vi "Cycling_No_DAQ_Tasks_RT - cOver100.vi"() -> ()   [LabVIEW 2020]
uses:
  Device-Interface-Layer/stop button3.vi
  Device-Interface-Layer/stop button2.vi
  Device-Interface-Layer/stop button1.vi
panel:
  out "Battery 1 Temp":dbl(graph)
  out "Battery 1 Strain":dbl(graph)
  out "Battery 1 Voltage":dbl(graph)
  out "Battery 1 Current":dbl(graph)
  out "Battery 2 Temp":dbl(graph)
  out "Battery 2 Strain":dbl(graph)
  out "Battery 2 Voltage":dbl(graph)
  out "Battery 2 Current":dbl(graph)
  out "Battery 3 Current":dbl(graph)
  out "Battery 3 Voltage":dbl(graph)
  out "Battery 3 Strain":dbl(graph)
  out "Boolean":bool=TRUE
  out "Battery 3 Temp":dbl(graph)
  out "PS Visa Out 3":refnum<visa-resource-name>
  out "PS error out 3":errorcluster
  in  "PS error in 3":errorcluster caption="PS error in (no error)"
  out "PS Visa Out 2":refnum<visa-resource-name>
  out "PS error out 2":errorcluster
  in  "PS error in 2":errorcluster caption="PS error in (no error)"
  out "PS error out":errorcluster
  out "PS Visa Out":refnum<visa-resource-name>
  in  "PS error in":errorcluster caption="PS error in (no error)"
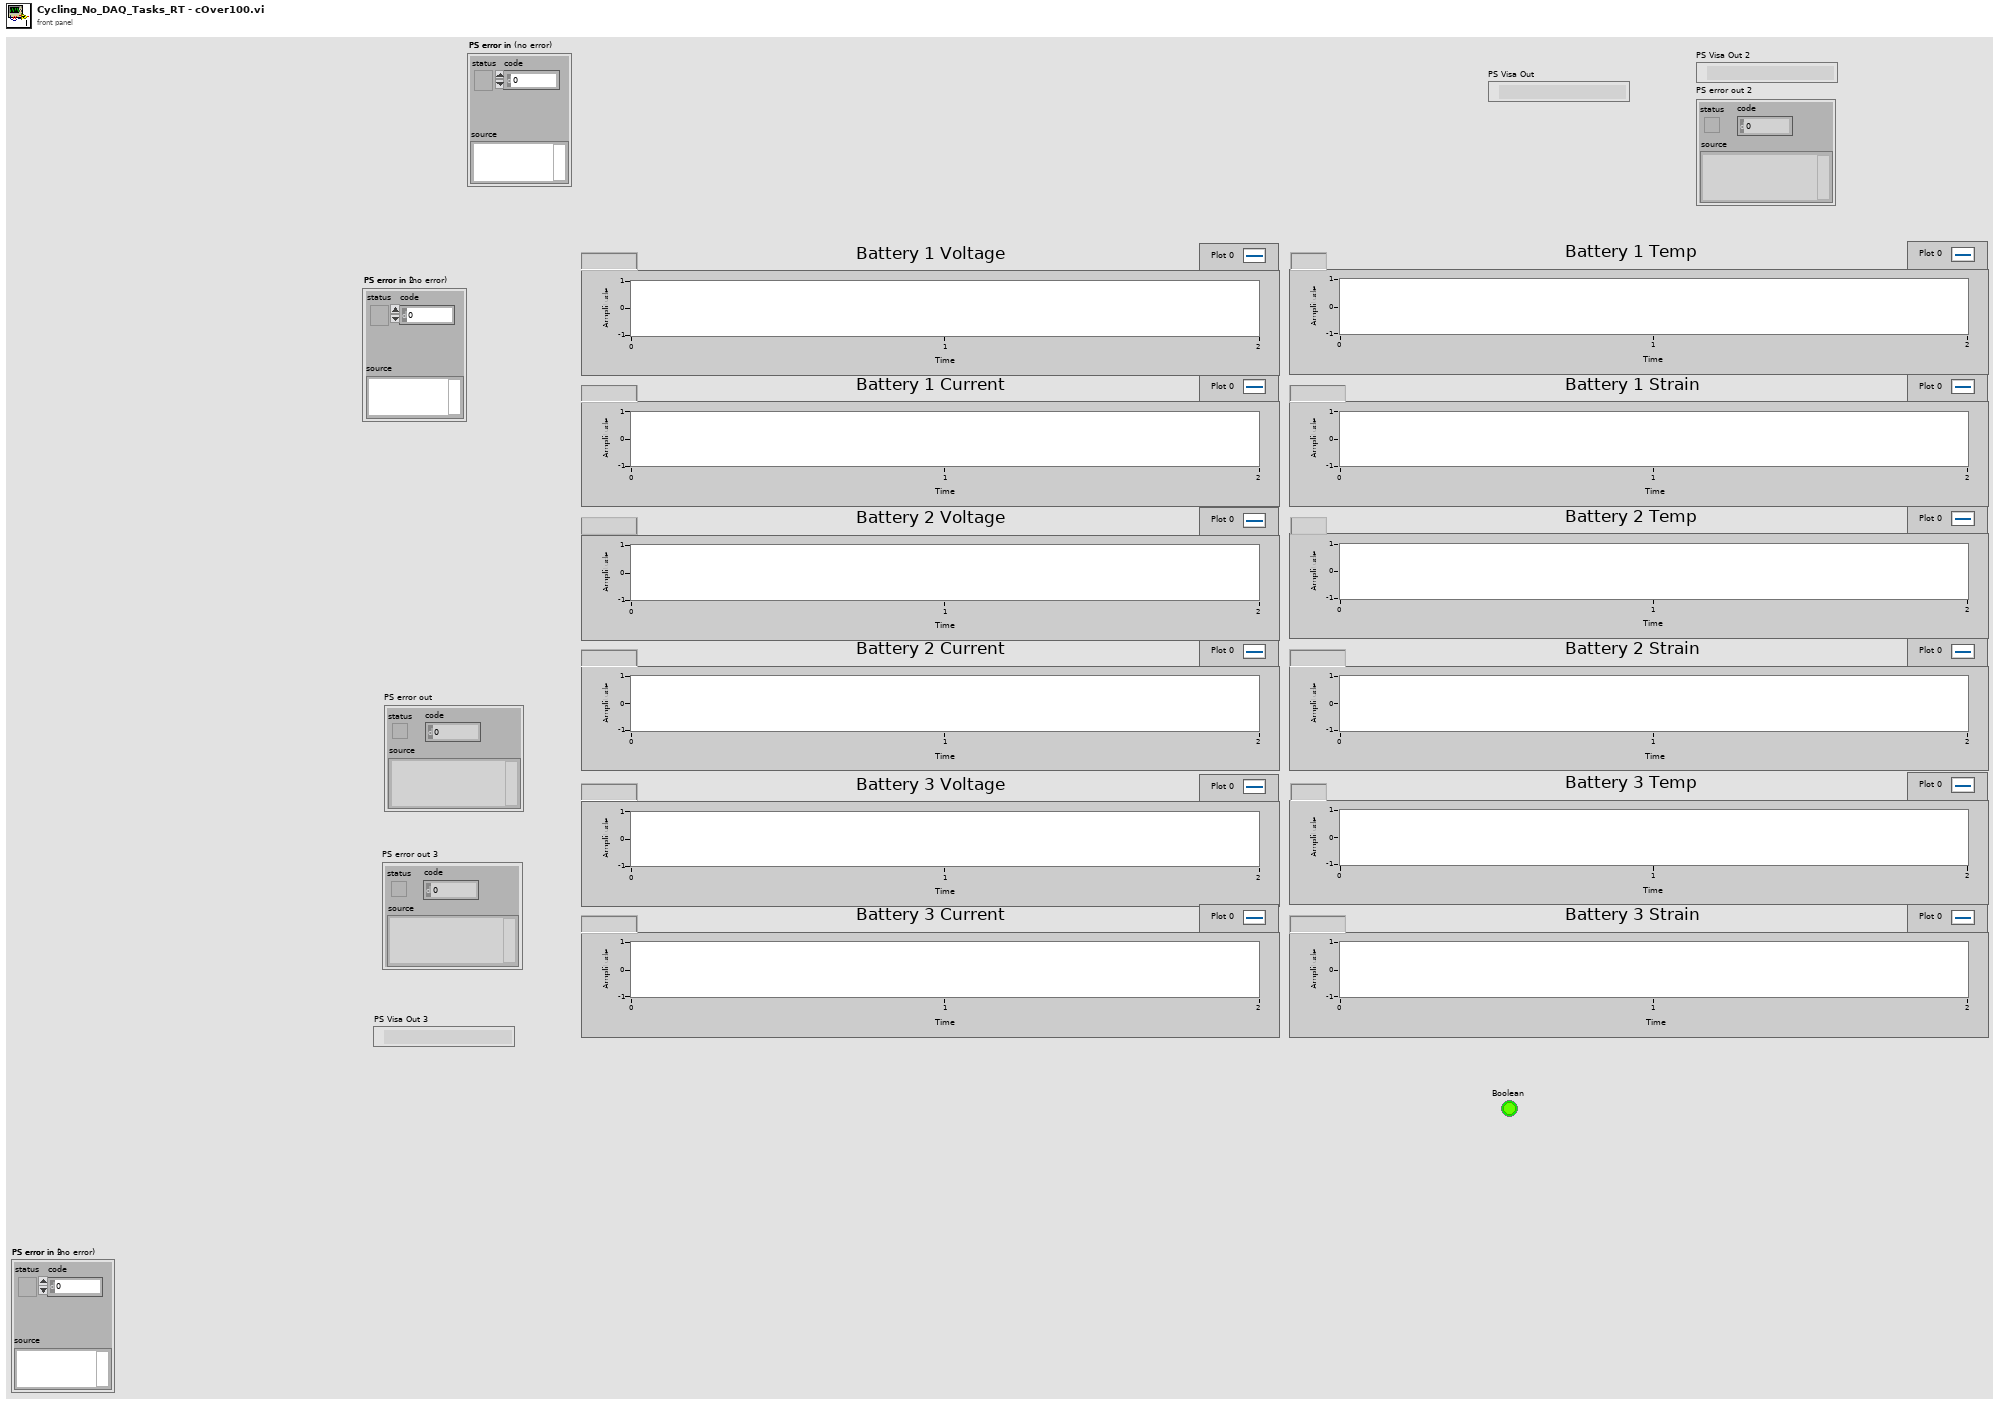
[diagram p1: front panel]
types:
  T1 = enum16{"\"30Q\"", "\"40T\"", "\"2P30Q\"", "\"3P30Q\"", "\"Nissan Leaf\""}
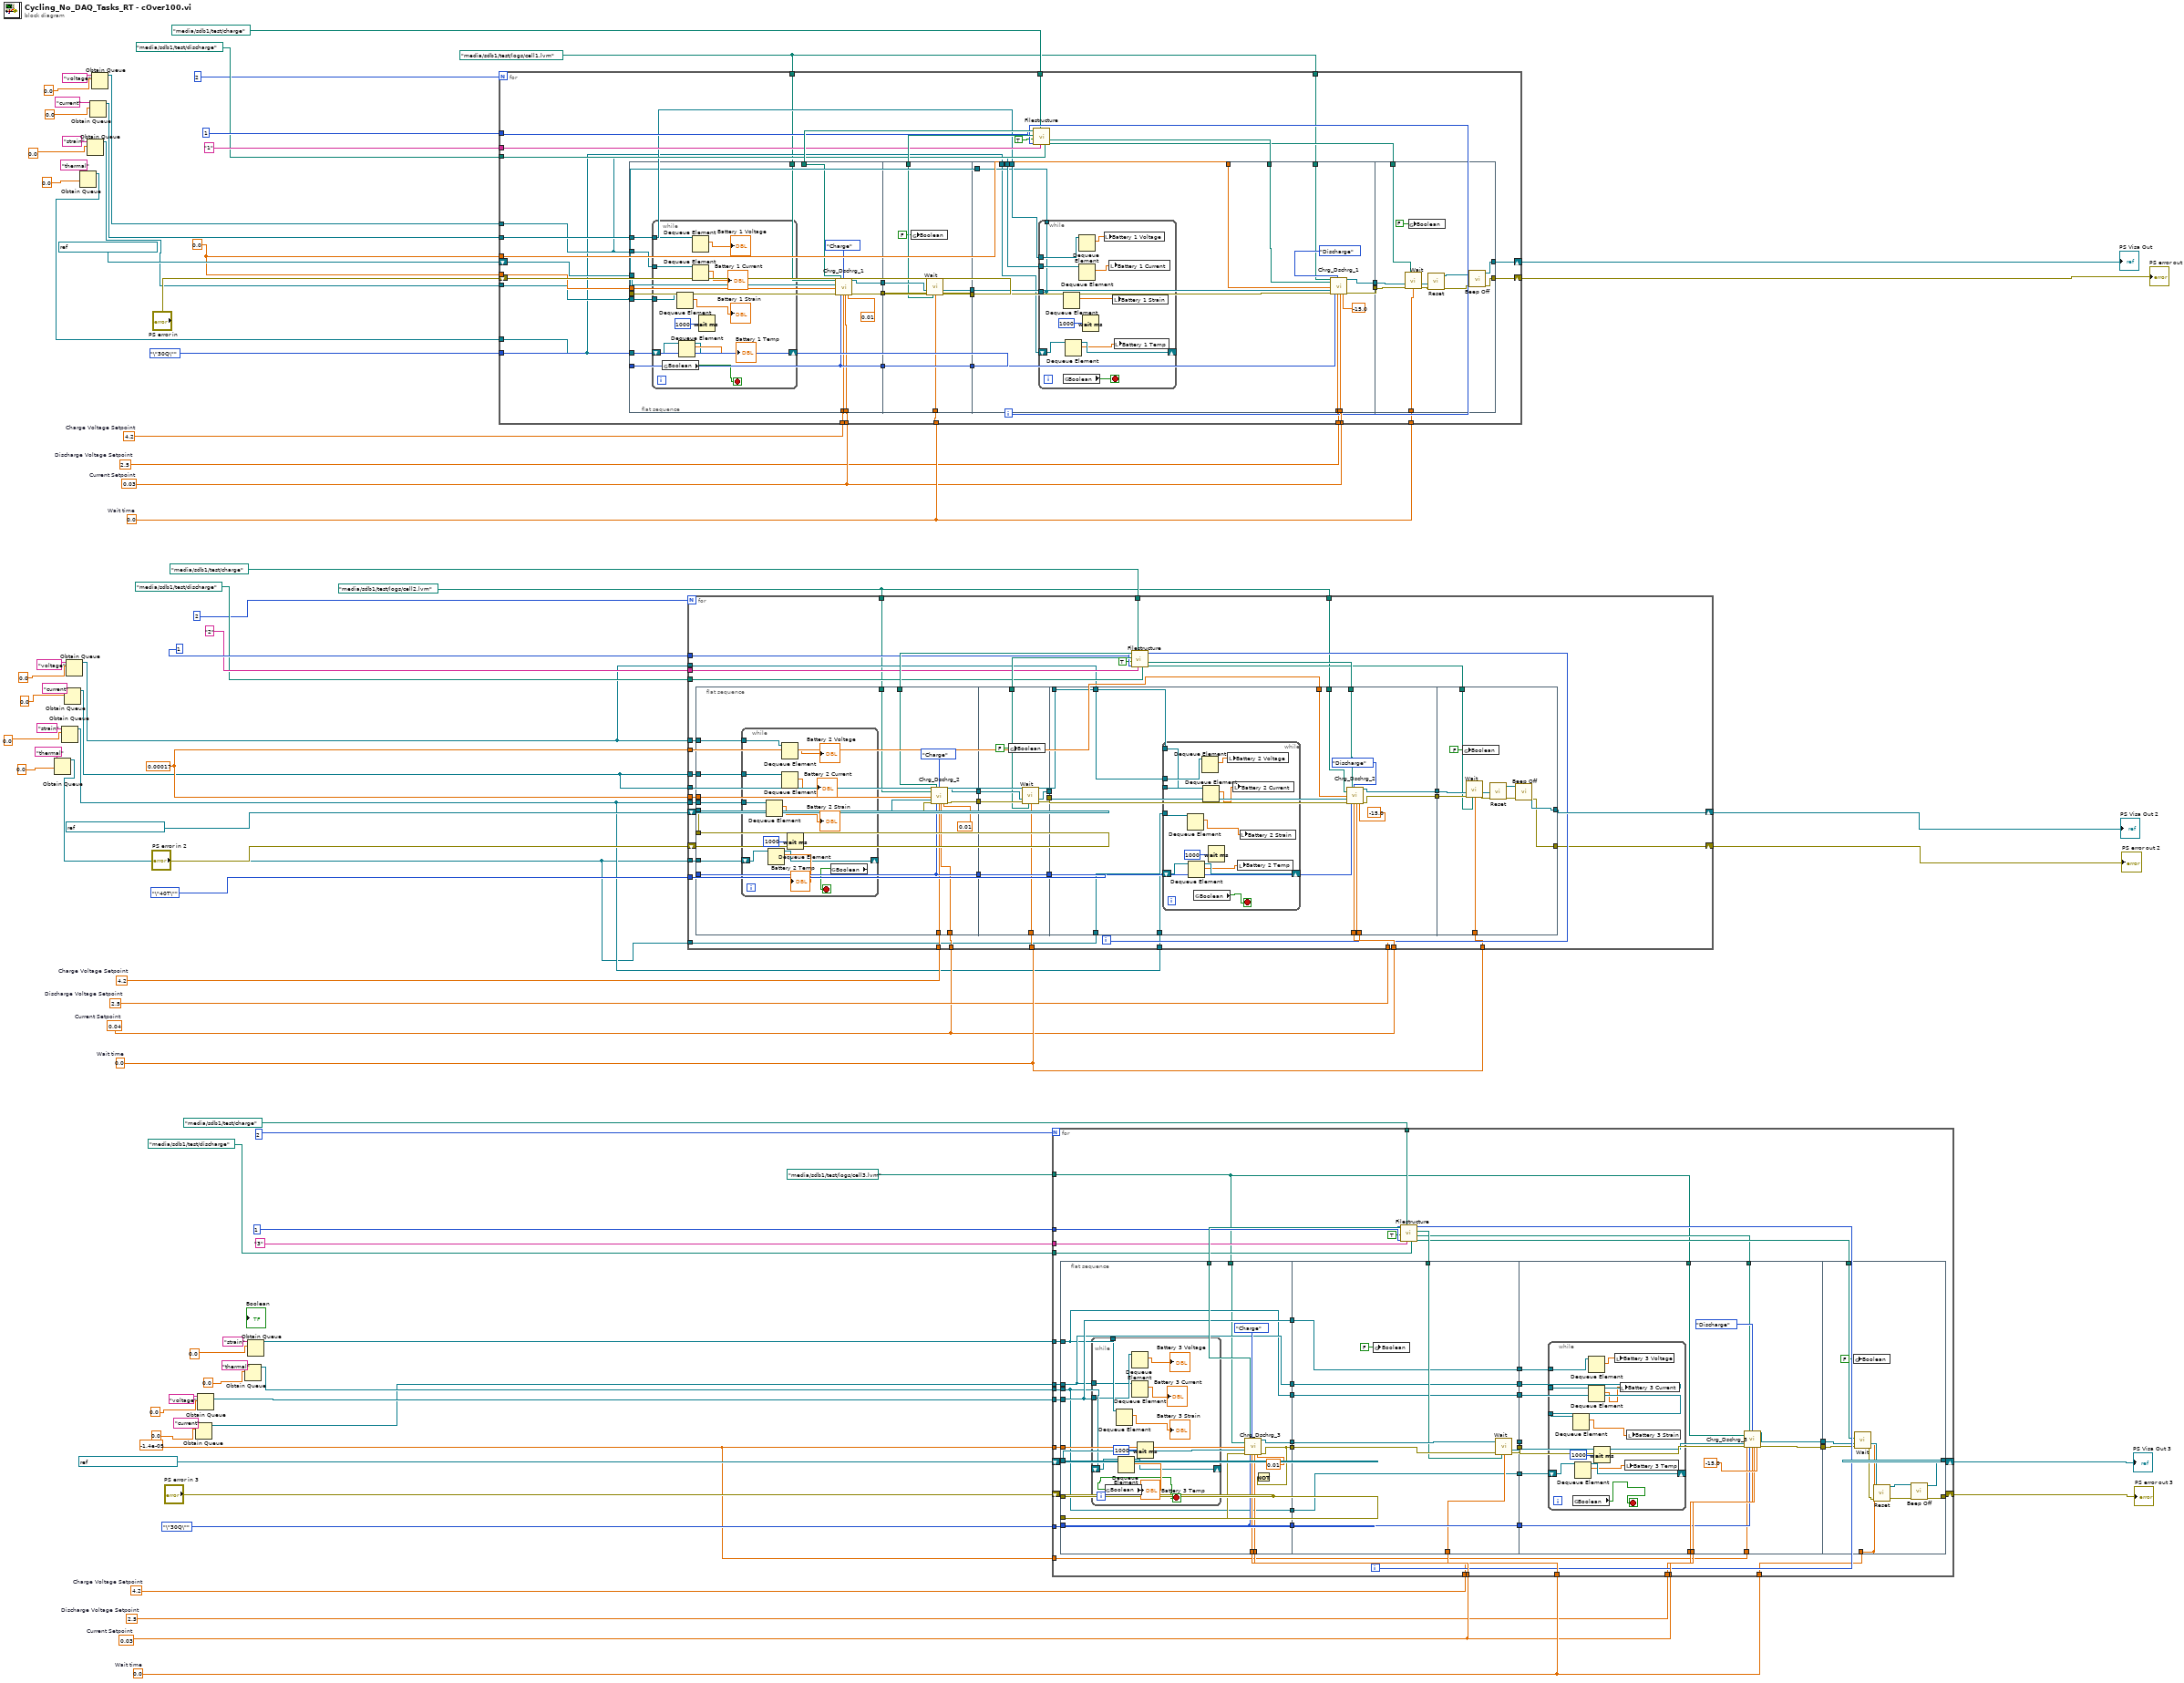
[diagram p0: block diagram]
diagram:
  w2 = path "/media/sdb1/test/logs/cell2.lvm" ("Error log filepath")
  w3 = path "/media/sdb1/test/logs/cell1.lvm" ("Error log filepath")
  w6 = -1.4e-05 ("Strain Offset")
  w41 = 0.00017 ("Strain Offset")
  w42 = 2.5  # Discharge Voltage Setpoint
  w45 = 0.0  # Wait time
  w43 = 0.03  # Current Setpoint
  w44 = 4.2  # Charge Voltage Setpoint
  w48 = 2.5  # Discharge Voltage Setpoint
  w49 = 0.0  # Wait time
  w47 = 0.04  # Current Setpoint
  w46 = 4.2  # Charge Voltage Setpoint
  w50 = 2.5  # Discharge Voltage Setpoint
  w53 = 0.0 ("Strain Offset")
  w54 = 0.0  # Wait time
  w52 = 0.03  # Current Setpoint
  w51 = 4.2  # Charge Voltage Setpoint
  n1 = Obtain Queue(name (unnamed)="thermal", element data type=0.0) -> (queue out=w7:refnum<queue>)  [unwired: 3 in, 2 out]
  n2 = Obtain Queue(name (unnamed)="strain", element data type=0.0) -> (queue out=w8:refnum<queue>)  [unwired: 3 in, 2 out]
  n3 = Obtain Queue(name (unnamed)="current", element data type=0.0) -> (queue out=w9:refnum<queue>)  [unwired: 3 in, 2 out]
  n4 = Obtain Queue(name (unnamed)="voltage", element data type=0.0) -> (queue out=w10:refnum<queue>)  [unwired: 3 in, 2 out]
  n5 = Obtain Queue(name (unnamed)="thermal", element data type=0.0) -> (queue out=w11:refnum<queue>)  [unwired: 3 in, 2 out]
  n6 = Obtain Queue(name (unnamed)="strain", element data type=0.0) -> (queue out=w12:refnum<queue>)  [unwired: 3 in, 2 out]
  n7 = Obtain Queue(name (unnamed)="current", element data type=0.0) -> (queue out=w13:refnum<queue>)  [unwired: 3 in, 2 out]
  n8 = Obtain Queue(name (unnamed)="voltage", element data type=0.0) -> (queue out=w14:refnum<queue>)  [unwired: 3 in, 2 out]
  n9 = Obtain Queue(name (unnamed)="current", element data type=0.0) -> (queue out=w33:refnum<queue>)  [unwired: 3 in, 2 out]
  n10 = Obtain Queue(name (unnamed)="voltage", element data type=0.0) -> (queue out=w34:refnum<queue>)  [unwired: 3 in, 2 out]
  n11 = Obtain Queue(name (unnamed)="thermal", element data type=0.0) -> (queue out=w39:refnum<queue>)  [unwired: 3 in, 2 out]
  n12 = Obtain Queue(name (unnamed)="strain", element data type=0.0) -> (queue out=w37:refnum<queue>)  [unwired: 3 in, 2 out]
  n13 = for {
    N: 2 ("Number of Cycles") -> [_]
    tunnel: T1."\"30Q\"" ("Battery Type") -> [w111]
    tunnel: w51 -> [w110]
    tunnel: w52 -> [w109]
    tunnel: w54 -> [w97]
    shift-right: [w88] -> w81
    shift-left: refnum<visa-resource-name> "TCPIP0::192.168.0.246::inst0::INSTR" ("PS VISA in") -> [w113]
    shift-right: [w87] -> w82
    shift-left: "PS error in" -> [w112]
    tunnel: 1 ("Starting Cycle") -> [w103]
    tunnel: "1" ("Batteryname") -> [w101]
    tunnel: path "/media/sdb1/test/discharge" ("Discharge filepath") -> [w100]
    tunnel: path "/media/sdb1/test/charge" ("Charge filepath") -> [w99]
    tunnel: w54 -> [w98]
    tunnel: w53 -> [w96]
    tunnel: w53 -> [w95]
    tunnel: w52 -> [w94]
    tunnel: w50 -> [w93]
    tunnel: w14 -> [w92]
    tunnel: w13 -> [w91]
    tunnel: w12 -> [w90]
    tunnel: w11 -> [w89]
    tunnel: w3 -> [w86]
    tunnel: w3 -> [w85]
    i -> [w104]
    n14 = flat-sequence {
      tunnel: w113 -> [w131]
      tunnel: w112 -> [w132]
      tunnel: w111 -> [w133]
      tunnel: w110 -> [w128]
      tunnel: [w135] -> w121
      tunnel: [w127] -> w120
      tunnel: [w133] -> w119
      tunnel: w108 -> [w136]
      tunnel: w96 -> [w130]
      tunnel: w94 -> [w129]
      tunnel: w92 -> [w126]
      tunnel: w91 -> [w125]
      tunnel: w90 -> [w124]
      tunnel: w89 -> [w123]
      tunnel: w86 -> [w122]
      tunnel: w121 -> [w155]
      tunnel: w120 -> [w154]
      tunnel: [w151] -> w118
      tunnel: [w152] -> w117
      tunnel: w119 -> [w156]
      tunnel: [w156] -> w116
      tunnel: w107 -> [w153]
      tunnel: w97 -> [w150]
      tunnel: w118 -> [w167]
      tunnel: w117 -> [w168]
      tunnel: w116 -> [w169]
      tunnel: w93 -> [w170]
      tunnel: w109 -> [w171]
      tunnel: w106 -> [w166]
      tunnel: [w164] -> w115
      tunnel: [w163] -> w114
      tunnel: w95 -> [w162]
      tunnel: w92 -> [w161]
      tunnel: w91 -> [w160]
      tunnel: w90 -> [w159]
      tunnel: w89 -> [w158]
      tunnel: w85 -> [w157]
      tunnel: w105 -> [w189]
      tunnel: w115 -> [w194]
      tunnel: w114 -> [w193]
      tunnel: w98 -> [w190]
      tunnel: [w185] -> w88
      tunnel: [w184] -> w87
      frame #0 {
        n15 = while {
          shift-right: [w146] -> _
          shift-left: w123 -> [w145]
          tunnel: w125 -> [w143]
          tunnel: w126 -> [w140]
          tunnel: w124 -> [w139]
          stop <- w138 stop-if-true
          n16 = global read "stop button1.vi" "Boolean"() -> (w138:bool)
          n17 = Dequeue Element(queue=w139) -> (element=→"Battery 1 Strain":dbl)  [unwired: 2 in, 3 out]
          n18 = Dequeue Element(queue=w145) -> (queue out=w146:refnum<queue>, element=→"Battery 1 Temp":dbl)  [unwired: 2 in, 2 out]
          n19 = Dequeue Element(queue=w140) -> (element=→"Battery 1 Voltage":dbl)  [unwired: 2 in, 3 out]
          n20 = Dequeue Element(queue=w143) -> (element=→"Battery 1 Current":dbl)  [unwired: 2 in, 3 out]
          n21 = Wait (ms)(milliseconds to wait=1000) -> ()  [unwired: 1 out]
        }
        n22 = call "Chrg_Dschrg_1.vi"("Error log filepath"=w122, "Strain Offset"=w130, "PS VISA in"=w131, "PS error in"=w132, "CyclePath"=w136, "Battery Type"=w133, "Charge/discharge"=enum8{"Charge", "Discharge"}."Charge", "Charge/Discharge Voltage Setpoint"=w128, "Current Setpoint"=w129, "Current Cutoff"=0.01) -> ("PS VISA out"=w135:refnum<visa-resource-name>, "PS error out"=w127:errorcluster)  [unwired: 8 in]
      }
      frame #1 {
        n23 = global write "stop button1.vi" "Boolean"(FALSE ("Boolean")) -> ()
        n24 = call "Wait.vi"("PS VISA in"=w155, "PS error in"=w154, "Wait Filepath"=w153, "Wait time"=w150) -> ("PS Visa Out"=w151:refnum<visa-resource-name>, "PS error out"=w152:errorcluster)  [unwired: 10 in]
      }
      frame #2 {
        n25 = while {
          shift-right: [w182] -> _
          shift-left: w158 -> [w181]
          tunnel: [w174] -> _
          tunnel: w160 -> [w180]
          tunnel: w161 -> [w175]
          tunnel: w159 -> [w174]
          stop <- w173 stop-if-true
          n26 = Dequeue Element(queue=w174) -> (element=w177:dbl)  [unwired: 2 in, 3 out]
          n27 = global read "stop button1.vi" "Boolean"() -> (w173:bool)
          n28 = Dequeue Element(queue=w181) -> (queue out=w182:refnum<queue>, element=w176:dbl)  [unwired: 2 in, 2 out]
          n29 = Dequeue Element(queue=w175) -> (element=w179:dbl)  [unwired: 2 in, 3 out]
          n30 = Dequeue Element(queue=w180) -> (element=w178:dbl)  [unwired: 2 in, 3 out]
          n31 = Wait (ms)(milliseconds to wait=1000) -> ()  [unwired: 1 out]
          n32 = local write "Battery 1 Voltage"(w179) -> ()
          n33 = local write "Battery 1 Current"(w178) -> ()
          n34 = local write "Battery 1 Strain"(w177) -> ()
          n35 = local write "Battery 1 Temp"(w176) -> ()
        }
        n36 = call "Chrg_Dschrg_1.vi"("Error log filepath"=w157, "Strain Offset"=w162, "PS VISA in"=w167, "PS error in"=w168, "CyclePath"=w166, "Battery Type"=w169, "Charge/discharge"=enum8{"Charge", "Discharge"}."Discharge", "Charge/Discharge Voltage Setpoint"=w170, "Current Setpoint"=w171, "Current Cutoff"=-15.0) -> ("PS VISA out"=w164:refnum<visa-resource-name>, "PS error out"=w163:errorcluster)  [unwired: 8 in]
      }
      frame #3 {
        n37 = call "Wait.vi"("PS VISA in"=w194, "PS error in"=w193, "Wait Filepath"=w189, "Wait time"=w190) -> ("PS Visa Out"=w192:refnum<visa-resource-name>, "PS error out"=w191:errorcluster)  [unwired: 10 in]
        n38 = global write "stop button1.vi" "Boolean"(FALSE ("Boolean")) -> ()
        n39 = call "Reset.vi"("error in"=w191, "VISA resource name"=w192) -> ("error out"=w186:errorcluster, "VISA resource name out"=w187:refnum<visa-resource-name>)  [unwired: 8 in]
        n40 = call "Beep Off.vi"("error in"=w186, "VISA resource name"=w187) -> ("error out"=w184:errorcluster, "VISA resource name out"=w185:refnum<visa-resource-name>)  [unwired: 8 in]
      }
    }
    n41 = call "Filestructure.vi"("Discharge filepath"=w100, "Batteryname"=w101, "Charge filepath"=w99, "For loop i"=w104, "In for loop"=TRUE, "Starting Cycle"=w103) -> ("DischargeWaitPath"=w105:path, "DischargeCyclePath"=w106:path, "ChargeWaitPath"=w107:path, "ChargeCyclePath"=w108:path)  [unwired: 1 in, 1 out]
  }
  "PS error out" <- w82
  "PS Visa Out" <- w81
  n42 = for {
    N: 2 ("Number of Cycles") -> [_]
    tunnel: T1."\"40T\"" ("Battery Type") -> [w225]
    tunnel: w47 -> [w224]
    tunnel: w47 -> [w223]
    shift-right: [w218] -> w71
    shift-left: refnum<visa-resource-name> "TCPIP0::192.168.0.247::inst0::INSTR" ("PS VISA in") -> [w227]
    shift-right: [w211] -> w72
    shift-left: "PS error in 2" -> [w226]
    tunnel: 1 ("Starting Cycle") -> [w216]
    tunnel: "2" ("Batteryname 2") -> [w214]
    tunnel: path "/media/sdb1/test/discharge" ("Discharge filepath") -> [w213]
    tunnel: path "/media/sdb1/test/charge" ("Charge filepath") -> [w212]
    tunnel: w49 -> [w210]
    tunnel: w49 -> [w209]
    tunnel: w48 -> [w208]
    tunnel: w46 -> [w207]
    tunnel: w41 -> [w206]
    tunnel: w41 -> [w205]
    tunnel: w10 -> [w204]
    tunnel: w9 -> [w203]
    tunnel: w8 -> [w202]
    tunnel: w7 -> [w201]
    tunnel: w10 -> [w200]
    tunnel: w9 -> [w199]
    tunnel: w8 -> [w198]
    tunnel: w7 -> [w197]
    tunnel: w2 -> [w196]
    tunnel: w2 -> [w195]
    i -> [w217]
    n43 = flat-sequence {
      tunnel: w227 -> [w245]
      tunnel: w226 -> [w246]
      tunnel: w225 -> [w247]
      tunnel: w224 -> [w248]
      tunnel: [w244] -> w235
      tunnel: [w241] -> w234
      tunnel: [w247] -> w233
      tunnel: w222 -> [w250]
      tunnel: w207 -> [w243]
      tunnel: w206 -> [w242]
      tunnel: w204 -> [w240]
      tunnel: w203 -> [w239]
      tunnel: w202 -> [w238]
      tunnel: w201 -> [w237]
      tunnel: w196 -> [w236]
      tunnel: w235 -> [w269]
      tunnel: w234 -> [w268]
      tunnel: [w264] -> w232
      tunnel: [w265] -> w231
      tunnel: w233 -> [w270]
      tunnel: [w270] -> w230
      tunnel: w221 -> [w267]
      tunnel: w209 -> [w266]
      tunnel: w232 -> [w281]
      tunnel: w231 -> [w282]
      tunnel: w230 -> [w283]
      tunnel: w208 -> [w284]
      tunnel: w223 -> [w285]
      tunnel: w220 -> [w280]
      tunnel: [w278] -> w229
      tunnel: [w277] -> w228
      tunnel: w205 -> [w276]
      tunnel: w200 -> [w275]
      tunnel: w199 -> [w274]
      tunnel: w198 -> [w273]
      tunnel: w197 -> [w272]
      tunnel: w195 -> [w271]
      tunnel: w219 -> [w303]
      tunnel: w229 -> [w308]
      tunnel: w228 -> [w307]
      tunnel: w210 -> [w304]
      tunnel: [w301] -> w218
      tunnel: [w298] -> w211
      frame #0 {
        n44 = while {
          shift-right: [w260] -> _
          shift-left: w237 -> [w259]
          tunnel: w239 -> [w257]
          tunnel: w240 -> [w254]
          tunnel: w238 -> [w253]
          stop <- w252 stop-if-true
          n45 = Dequeue Element(queue=w253) -> (element=→"Battery 2 Strain":dbl)  [unwired: 2 in, 3 out]
          n46 = Dequeue Element(queue=w259) -> (queue out=w260:refnum<queue>, element=→"Battery 2 Temp":dbl)  [unwired: 2 in, 2 out]
          n47 = Dequeue Element(queue=w254) -> (element=→"Battery 2 Voltage":dbl)  [unwired: 2 in, 3 out]
          n48 = Dequeue Element(queue=w257) -> (element=→"Battery 2 Current":dbl)  [unwired: 2 in, 3 out]
          n49 = Wait (ms)(milliseconds to wait=1000) -> ()  [unwired: 1 out]
          n50 = global read "stop button2.vi" "Boolean"() -> (w252:bool)
        }
        n51 = call "Chrg_Dschrg_2.vi"("Error log filepath"=w236, "Strain Offset"=w242, "PS VISA in"=w245, "PS error in"=w246, "CyclePath"=w250, "Battery Type"=w247, "Charge/discharge"=enum8{"Charge", "Discharge"}."Charge", "Charge/Discharge Voltage Setpoint"=w243, "Current Setpoint"=w248, "Current Cutoff"=0.01) -> ("PS VISA out"=w244:refnum<visa-resource-name>, "PS error out"=w241:errorcluster)  [unwired: 8 in]
      }
      frame #1 {
        n52 = global write "stop button2.vi" "Boolean"(FALSE ("Boolean")) -> ()
        n53 = call "Wait.vi"("PS VISA in"=w269, "PS error in"=w268, "Wait Filepath"=w267, "Wait time"=w266) -> ("PS Visa Out"=w264:refnum<visa-resource-name>, "PS error out"=w265:errorcluster)  [unwired: 10 in]
      }
      frame #2 {
        n54 = while {
          shift-right: [w296] -> _
          shift-left: w272 -> [w295]
          tunnel: w273 -> [w294]
          tunnel: [w288] -> _
          tunnel: w275 -> [w289]
          tunnel: w274 -> [w288]
          stop <- w287 stop-if-true
          n55 = Dequeue Element(queue=w294) -> (element=w291:dbl)  [unwired: 2 in, 3 out]
          n56 = Dequeue Element(queue=w295) -> (queue out=w296:refnum<queue>, element=w290:dbl)  [unwired: 2 in, 2 out]
          n57 = global read "stop button2.vi" "Boolean"() -> (w287:bool)
          n58 = Dequeue Element(queue=w289) -> (element=w293:dbl)  [unwired: 2 in, 3 out]
          n59 = Dequeue Element(queue=w288) -> (element=w292:dbl)  [unwired: 2 in, 3 out]
          n60 = Wait (ms)(milliseconds to wait=1000) -> ()  [unwired: 1 out]
          n61 = local write "Battery 2 Voltage"(w293) -> ()
          n62 = local write "Battery 2 Current"(w292) -> ()
          n63 = local write "Battery 2 Temp"(w290) -> ()
          n64 = local write "Battery 2 Strain"(w291) -> ()
        }
        n65 = call "Chrg_Dschrg_2.vi"("Error log filepath"=w271, "Strain Offset"=w276, "PS VISA in"=w281, "PS error in"=w282, "CyclePath"=w280, "Battery Type"=w283, "Charge/discharge"=enum8{"Charge", "Discharge"}."Discharge", "Charge/Discharge Voltage Setpoint"=w284, "Current Setpoint"=w285, "Current Cutoff"=-15.0) -> ("PS VISA out"=w278:refnum<visa-resource-name>, "PS error out"=w277:errorcluster)  [unwired: 8 in]
      }
      frame #3 {
        n66 = global write "stop button2.vi" "Boolean"(FALSE ("Boolean")) -> ()
        n67 = call "Wait.vi"("PS VISA in"=w308, "PS error in"=w307, "Wait Filepath"=w303, "Wait time"=w304) -> ("PS Visa Out"=w306:refnum<visa-resource-name>, "PS error out"=w305:errorcluster)  [unwired: 10 in]
        n68 = call "Reset.vi"("error in"=w305, "VISA resource name"=w306) -> ("error out"=w299:errorcluster, "VISA resource name out"=w300:refnum<visa-resource-name>)  [unwired: 8 in]
        n69 = call "Beep Off.vi"("error in"=w299, "VISA resource name"=w300) -> ("error out"=w298:errorcluster, "VISA resource name out"=w301:refnum<visa-resource-name>)  [unwired: 8 in]
      }
    }
    n70 = call "Filestructure.vi"("Discharge filepath"=w213, "Batteryname"=w214, "Charge filepath"=w212, "For loop i"=w217, "In for loop"=TRUE, "Starting Cycle"=w216) -> ("DischargeWaitPath"=w219:path, "DischargeCyclePath"=w220:path, "ChargeWaitPath"=w221:path, "ChargeCyclePath"=w222:path)  [unwired: 1 in, 1 out]
  }
  "PS error out 2" <- w72
  "PS Visa Out 2" <- w71
  n71 = for {
    N: 2 ("Number of Cycles") -> [_]
    tunnel: T1."\"30Q\"" ("Battery Type") -> [w343]
    tunnel: w43 -> [w342]
    tunnel: w43 -> [w341]
    tunnel: w45 -> [w337]
    shift-right: [w336] -> w61
    shift-left: refnum<visa-resource-name> "TCPIP0::192.168.0.248::inst0::INSTR" ("PS VISA in") -> [w344]
    shift-right: [w329] -> w62
    shift-left: "PS error in 3" -> [w324]
    tunnel: 1 ("Starting Cycle") -> [w334]
    tunnel: "3" ("Batteryname 3") -> [w332]
    tunnel: path "/media/sdb1/test/discharge" ("Discharge filepath") -> [w331]
    tunnel: path "/media/sdb1/test/charge" ("Charge filepath") -> [w330]
    tunnel: w45 -> [w328]
    tunnel: w44 -> [w327]
    tunnel: w42 -> [w326]
    tunnel: w6 -> [w325]
    tunnel: w39 -> [w323]
    tunnel: w37 -> [w322]
    tunnel: w34 -> [w321]
    tunnel: w33 -> [w320]
    tunnel: w6 -> [w311]
    tunnel: path "/media/sdb1/test/logs/cell3.lvm" ("Error log filepath") -> [w309]
    i -> [w335]
    n72 = flat-sequence {
      tunnel: w344 -> [w361]
      tunnel: w324 -> [w362]
      tunnel: w343 -> [w363]
      tunnel: w342 -> [w364]
      tunnel: [w366] -> w352
      tunnel: [w358] -> w351
      tunnel: [w363] -> w350
      tunnel: w340 -> [w367]
      tunnel: w327 -> [w360]
      tunnel: w325 -> [w359]
      tunnel: w324 -> [_]
      tunnel: w323 -> [w354]
      tunnel: w322 -> [w355]
      tunnel: w321 -> [w357]
      tunnel: w320 -> [w356]
      tunnel: [w357] -> w319
      tunnel: [w356] -> w318
      tunnel: [w355] -> w317
      tunnel: [w354] -> w316
      tunnel: w309 -> [w353]
      tunnel: w352 -> [w390]
      tunnel: w351 -> [w389]
      tunnel: [w380] -> w349
      tunnel: [w386] -> w348
      tunnel: w350 -> [w391]
      tunnel: [w391] -> w347
      tunnel: w339 -> [w388]
      tunnel: w337 -> [w387]
      tunnel: w319 -> [w385]
      tunnel: w318 -> [w384]
      tunnel: w317 -> [w383]
      tunnel: w316 -> [w382]
      tunnel: [w385] -> w315
      tunnel: [w384] -> w314
      tunnel: [w383] -> w313
      tunnel: [w382] -> w312
      tunnel: w349 -> [w402]
      tunnel: w348 -> [w403]
      tunnel: w347 -> [w404]
      tunnel: w326 -> [w405]
      tunnel: w341 -> [w406]
      tunnel: [w400] -> w346
      tunnel: [w399] -> w345
      tunnel: w315 -> [w398]
      tunnel: w314 -> [w397]
      tunnel: w313 -> [w396]
      tunnel: w312 -> [w395]
      tunnel: w311 -> [w394]
      tunnel: w310 -> [w393]
      tunnel: w309 -> [w392]
      tunnel: w338 -> [w425]
      tunnel: w346 -> [w429]
      tunnel: w345 -> [w428]
      tunnel: [w424] -> _
      tunnel: [w422] -> w336
      tunnel: [w419] -> w329
      tunnel: w328 -> [w424]
      frame #0 {
        n73 = while {
          shift-right: [w377] -> _
          shift-left: w354 -> [w376]
          tunnel: w355 -> [w375]
          tunnel: w357 -> [w373]
          tunnel: w356 -> [w372]
          stop <- w369 stop-if-true
          n74 = global read "stop button3.vi" "Boolean"() -> (w369:bool)
          n75 = Dequeue Element(queue=w375) -> (element=→"Battery 3 Strain":dbl)  [unwired: 2 in, 3 out]
          n76 = Dequeue Element(queue=w376) -> (queue out=w377:refnum<queue>, element=→"Battery 3 Temp":dbl)  [unwired: 2 in, 2 out]
          n77 = Dequeue Element(queue=w373) -> (element=→"Battery 3 Voltage":dbl)  [unwired: 2 in, 3 out]
          n78 = Dequeue Element(queue=w372) -> (element=→"Battery 3 Current":dbl)  [unwired: 2 in, 3 out]
          n79 = Wait (ms)(milliseconds to wait=1000) -> ()  [unwired: 1 out]
        }
        n80 = call "Chrg_Dschrg_3.vi"("Error log filepath"=w353, "Strain Offset"=w359, "PS VISA in"=w361, "PS error in"=w362, "CyclePath"=w367, "Battery Type"=w363, "Charge/discharge"=enum8{"Charge", "Discharge"}."Charge", "Charge/Discharge Voltage Setpoint"=w360, "Current Setpoint"=w364, "Current Cutoff"=0.01) -> ("PS VISA out"=w366:refnum<visa-resource-name>, "PS error out"=w358:errorcluster)  [unwired: 8 in]
        n81 = Not(x=w358) -> ()  [unwired: 1 out]
      }
      frame #1 {
        n82 = global write "stop button3.vi" "Boolean"(FALSE ("Boolean")) -> ()
        n83 = call "Wait.vi"("PS VISA in"=w390, "PS error in"=w389, "Wait Filepath"=w388, "Wait time"=w387) -> ("PS Visa Out"=w380:refnum<visa-resource-name>, "PS error out"=w386:errorcluster)  [unwired: 10 in]
      }
      frame #2 {
        n84 = while {
          shift-right: [w417] -> _
          shift-left: w395 -> [w416]
          tunnel: w396 -> [w415]
          tunnel: w397 -> [w414]
          tunnel: w398 -> [w409]
          stop <- w408 stop-if-true
          n85 = Dequeue Element(queue=w415) -> (element=w411:dbl)  [unwired: 2 in, 3 out]
          n86 = global read "stop button3.vi" "Boolean"() -> (w408:bool)
          n87 = Dequeue Element(queue=w416) -> (queue out=w417:refnum<queue>, element=w410:dbl)  [unwired: 2 in, 2 out]
          n88 = Dequeue Element(queue=w409) -> (element=w413:dbl)  [unwired: 2 in, 3 out]
          n89 = Dequeue Element(queue=w414) -> (element=w412:dbl)  [unwired: 2 in, 3 out]
          n90 = Wait (ms)(milliseconds to wait=1000) -> ()  [unwired: 1 out]
          n91 = local write "Battery 3 Voltage"(w413) -> ()
          n92 = local write "Battery 3 Current"(w412) -> ()
          n93 = local write "Battery 3 Temp"(w410) -> ()
          n94 = local write "Battery 3 Strain"(w411) -> ()
        }
        n95 = call "Chrg_Dschrg_3.vi"("Error log filepath"=w392, "Strain Offset"=w394, "PS VISA in"=w402, "PS error in"=w403, "CyclePath"=w393, "Battery Type"=w404, "Charge/discharge"=enum8{"Charge", "Discharge"}."Discharge", "Charge/Discharge Voltage Setpoint"=w405, "Current Setpoint"=w406, "Current Cutoff"=-15.0) -> ("PS VISA out"=w400:refnum<visa-resource-name>, "PS error out"=w399:errorcluster)  [unwired: 8 in]
      }
      frame #3 {
        n96 = global write "stop button3.vi" "Boolean"(FALSE ("Boolean")) -> ()
        n97 = call "Wait.vi"("PS VISA in"=w429, "PS error in"=w428, "Wait Filepath"=w425, "Wait time"=w424) -> ("PS Visa Out"=w427:refnum<visa-resource-name>, "PS error out"=w426:errorcluster)  [unwired: 10 in]
        n98 = call "Reset.vi"("error in"=w426, "VISA resource name"=w427) -> ("error out"=w420:errorcluster, "VISA resource name out"=w421:refnum<visa-resource-name>)  [unwired: 8 in]
        n99 = call "Beep Off.vi"("error in"=w420, "VISA resource name"=w421) -> ("error out"=w419:errorcluster, "VISA resource name out"=w422:refnum<visa-resource-name>)  [unwired: 8 in]
      }
    }
    n100 = call "Filestructure.vi"("Discharge filepath"=w331, "Batteryname"=w332, "Charge filepath"=w330, "For loop i"=w335, "In for loop"=TRUE, "Starting Cycle"=w334) -> ("DischargeWaitPath"=w338:path, "DischargeCyclePath"=w310:path, "ChargeWaitPath"=w339:path, "ChargeCyclePath"=w340:path)  [unwired: 1 in, 1 out]
  }
  "PS error out 3" <- w62
  "PS Visa Out 3" <- w61
